vi "IVI_Oscilloscope.vi"() -> ()   [LabVIEW 2013]
doc: "This example shows how to use autosetup and acquire a waveform on a single channel for acquiring waveforms in a loop until stopped by user."
uses:
  IVI_chan.ctl
  Global.vi
panel:
  out "SQUID":string="24"
  in  "stop":bool
  in  "Tab Control":T1(tab)
  out "Saving":bool
  out "Waveform Data":waveform(dbl)[](graph)=[{"t0"=timestamp(1.3199999999947629e-08 s since 1904-01-01), "dt"=1e-06, "Y"=array[1000 elements]}, {"t0"=timestamp(1.3199999999947629e-08 s since 1904-01-01), "dt"=1e-06, "Y"=array[1000 elements]}]
  out "Points":i32=1000
  out "dt":dbl=1e-06 format="%#_2e"
  out "Repeat":u32=117
  out "Manufacturer":string="TEKTRONIX"
  out "Model":string="TDS 3054"
  out "Stats":T2(array[cluster])=[{"Min"=-2.081126189757815, "t (min)"=0.00037999999999999997, "Max"=3.0405276847871723, "t (max)"=0.0006399999999999999, "Range"=5.121653874544988, "Mean"=0.4992700288991155, "Std"=1.7686679103049028}, {"Min"=-1.0, "t (min)"=0.00030199999999999997, "Max"=1.0, "t (max)"=1.7e-05, "Range"=2.0, "Mean"=0.13208653234179343, "Std"=0.8981746888230542}] {"t (min)" format="%#_6p"; "t (max)" format="%#_6p"}
  in  "trigger level":dbl format="%#_13g"
  in  "trigger slope":i32(ring)=1 items=["Positive"=1, "Negative"=0]
  in  "trigger coupling":i32(ring)=1 items=["AC"=0, "DC"=1, "HF Reject"=3, "LF Reject"=4, "Noise Reject"=5]
  in  "trigger source":string(combo)="CHANNEL1"
  out "error out":errorcluster
  in  "Channels":T3[](array[typedef])=[{"channel name"="CHANNEL1", "probe attenuation"=1.0, "vertical offset"=0.0, "vertical range"=10.0, "vertical coupling"=1, "input impedance"=1000000.0}, {"channel name"="CHANNEL2", "probe attenuation"=1.0, "vertical offset"=0.0, "vertical range"=2.0, "vertical coupling"=1, "input impedance"=1000000.0}] {"input impedance" format="%#_13g"; "vertical coupling" items=["AC", "DC", "GND"]; "vertical range" format="%.3f"; "vertical offset" format="%.3f"; "probe attenuation" format="%.3f"}
  in  "logical name":refnum<k15>="Scope" caption="IVI Oscilloscope"
  in  "time per record":dbl=0.001 format="%^.2e"
  in  "acquisition start time":dbl format="%.3f"
  in  "min record length":i32=1000
  in  "wait (ms)":u32=500
  in  "Bin size":i16=1
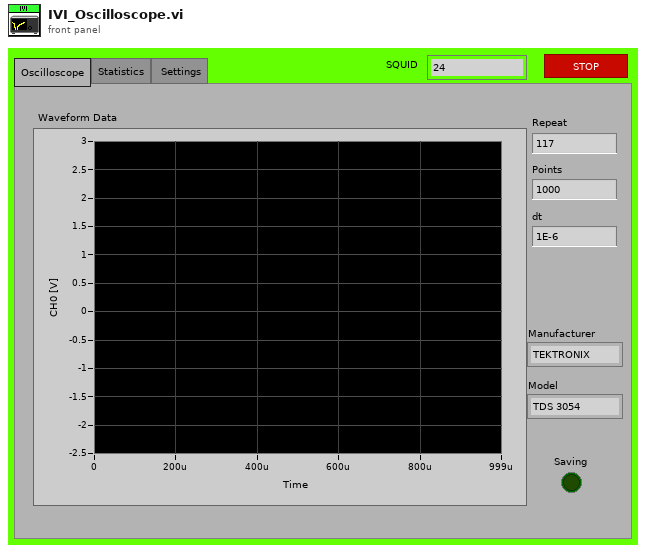
[diagram p1: front panel]
types:
  T1 = enum32{"Oscilloscope", "Statistics", " Settings"}
  T2 = cluster{"Min":dbl, "t (min)":dbl, "Max":dbl, "t (max)":dbl, "Range":dbl, "Mean":dbl, "Std":dbl}[]
  T3 = typedef "IVI_chan.ctl" = cluster{"channel name":string, "probe attenuation":dbl, "vertical offset":dbl, "vertical range":dbl, "vertical coupling":i32, "input impedance":dbl}
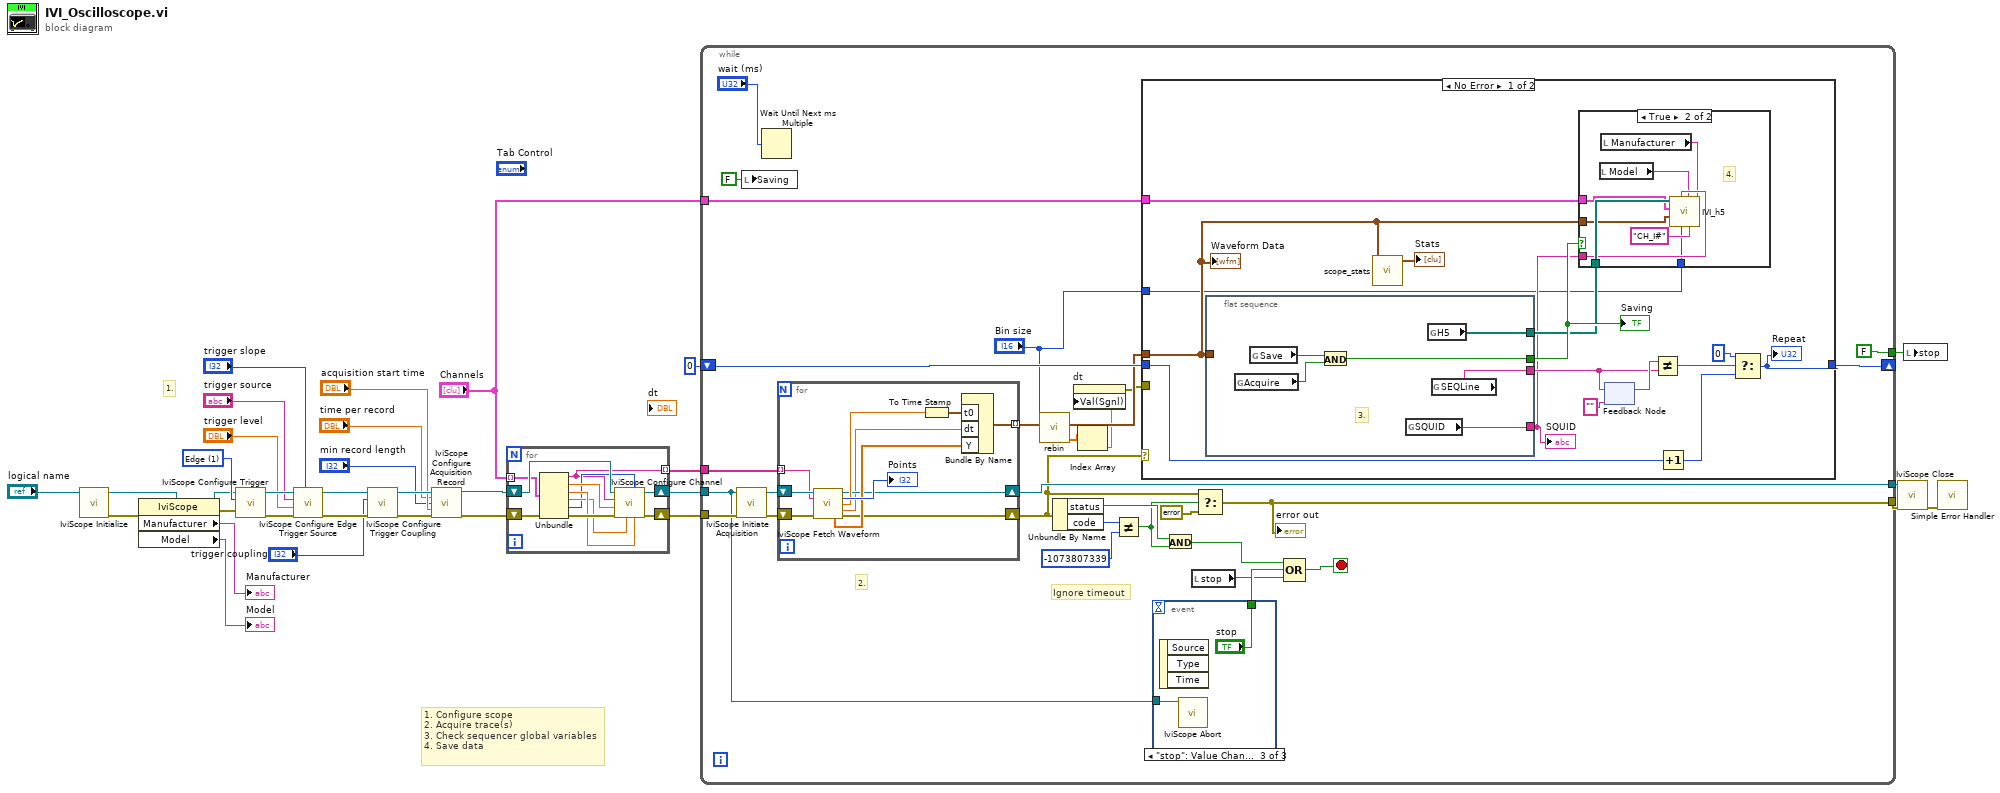
[diagram p0: block diagram]
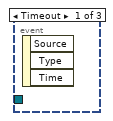
[diagram p2: hidden frame]
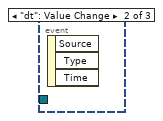
[diagram p3: hidden frame]
diagram:
  w29 = 1 items=["Edge"=1, "TV"=5, "Runt"=3, "Glitch"=4, "Width"=2, "AC Line"=7, "Immediate"=6] ("trigger type (Edge)")
  # "1."
  # "1. Configure scope\n2. Acquire trace(s)\n3. Check sequencer global variables\n4. Save data"
  n1 = call <vilib>:"IviScope Initialize.vi"("logical name (\"SampleScope\")"="logical name") -> ("error out"=w6:errorcluster, "instrument handle out"=w5:refnum<k15>)  [unwired: 9 in]
  n2 = property class="IviScope"(reference=w5, error in=w6) -> (reference out=w4:refnum<k15>, error out=w3:errorcluster, "Manufacturer"=→"Manufacturer":string, "Model"=→"Model":string)
  n3 = call <vilib>:"IviScope Configure Trigger.vi"("error in (no error)"=w3, "trigger type (Edge)"=w29, "instrument handle"=w4) -> ("error out"=w26:errorcluster, "instrument handle out"=w27:refnum<k15>)  [unwired: 7 in]
  n4 = call <vilib>:"IviScope Configure Edge Trigger Source.vi"("trigger slope (Positive)"="trigger slope", "error in (no error)"=w26, "trigger level  (0.0 V)"="trigger level", "trigger source (CHANNEL1)"="trigger source", "instrument handle"=w27) -> ("error out"=w25:errorcluster, "instrument handle out"=w28:refnum<k15>)  [unwired: 5 in]
  n5 = call <vilib>:"IviScope Configure Trigger Coupling.vi"("error in (no error)"=w25, "trigger coupling (DC)"="trigger coupling", "instrument handle"=w28) -> ("error out"=w24:errorcluster, "instrument handle out"=w23:refnum<k15>)  [unwired: 7 in]
  n6 = call <vilib>:"IviScope Configure Acquisition Record.vi"("instrument handle"=w23, "time per record (1.0E-3 s)"="time per record", "min record length (100 samples)"="min record length", "acquisition start time (0.0 s)"="acquisition start time", "error in (no error)"=w24) -> ("instrument handle out"=w20:refnum<k15>, "error out"=w21:errorcluster)  [unwired: 9 in]
  n7 = for {
    tunnel: "Channels" -> [w38] mode=indexing
    shift-right: [w42] -> w17
    shift-left: w20 -> [w39]
    shift-right: [w41] -> w16
    shift-left: w21 -> [w40]
    tunnel: [w33] -> w11 mode=indexing
    n8 = Unbundle(w38) -> ("channel name"=w33:string, "probe attenuation"=w37:dbl, "vertical offset"=w36:dbl, "vertical range"=w35:dbl, "vertical coupling"=w34:i32)  [unwired: 1 out]
    n9 = call <vilib>:"IviScope Configure Channel.vi"("vertical offset (0.0 V)"=w36, "vertical coupling (DC)"=w34, "vertical range (10.0 V)"=w35, "error in (no error)"=w40, "probe attenuation (1:1.0)"=w37, "channel name (\"CHANNEL1\")"=w33, "instrument handle"=w39) -> ("error out"=w41:errorcluster, "instrument handle out"=w42:refnum<k15>)  [unwired: 3 in]
  }
  n10 = while {
    tunnel: [w56] -> w10
    tunnel: [w63] -> w8
    shift-right: [w65] -> _
    shift-left: u32 0 ("millisecond multiple") -> [w66]
    tunnel: [FALSE ("stop")] -> w31
    tunnel: w17 -> [w52]
    tunnel: w16 -> [w60]
    tunnel: w11 -> [w57]
    tunnel: "Channels" -> [w54]
    stop <- w70 stop-if-true
    # "Ignore timeout"
    # "2."
    n11 = call <vilib>:"IviScope Initiate Acquisition.vi"("error in (no error)"=w60, "instrument handle"=w52) -> ("error out"=w58:errorcluster, "instrument handle out"=w59:refnum<k15>)  [unwired: 8 in]
    n12 = local write "Saving"(FALSE ("Saving")) -> ()
    n13 = Wait Until Next ms Multiple(millisecond multiple="wait (ms)") -> ()  [unwired: 1 out]
    n14 = for {
      tunnel: w57 -> [w81] mode=indexing
      tunnel: [w77] -> w47 mode=indexing
      shift-right: [w76] -> w56
      shift-left: w59 -> [w83]
      shift-right: [w74] -> w55
      shift-left: w58 -> [w84]
      n15 = call <vilib>:"IviScope Fetch Waveform.vi"("instrument handle"=w83, "channel name (\"CHANNEL1\")"=w81, "error in (no error)"=w84) -> ("instrument handle out"=w76:refnum<k15>, "actual points"=→"Points":i32, "initial x"=w78:dbl, "x increment"=w75:dbl, "waveform array"=w80:dbl[], "error out"=w74:errorcluster)  [unwired: 7 in]
      n16 = To Time Stamp(1:w78) -> (0:w79:timestamp)
      n17 = Bundle By Name("t0"=w79, "dt"=w75, "Y"=w80) -> (w77:waveform(dbl))  [unwired: 1 in]
    }
    n18 = call "rebin.vi"("Bin size"="Bin size", "Waveform Data IN"=w47) -> ("dt"=w45:dbl[], "Waveform Data OUT"=w48:waveform(dbl)[])  [unwired: 6 in, 1 out]
    n19 = Unbundle By Name(w55) -> ("status"=w67:bool, "code"=w69:i32)
    n20 = Index Array(array=w45) -> (element=w46:dbl)  [unwired: 1 in]
    n21 = property on="dt" class="DigNum (strict)"("Val(Sgnl)"=w46) -> (error out=w44:errorcluster)  [unwired: 2 in, 1 out]
    n22 = Not Equal?(x=w69, y=-1073807339) -> (x != y?=w64:bool)
    n23 = case shown="No Error" w55 {
      tunnel: w48 -> [w92 _]
      tunnel: w66 -> [w95 w114]
      tunnel: [w89 w114] -> w65
      tunnel: w54 -> [w91 _]
      tunnel: w44 -> [_ _]
      tunnel: "Bin size" -> [w85 _]
      frame No Error {
        n24 = flat-sequence {
          tunnel: w92 -> [_]
          tunnel: [w103] -> w90
          tunnel: [w102] -> w88
          tunnel: [w101] -> w87
          tunnel: [w100] -> w86
          frame #0 {
            # "3."
            n25 = global read "Global.vi" "Acquire"() -> (w105:bool)
            n26 = global read "Global.vi" "Save"() -> (w104:bool)
            n27 = And(x=w104, y=w105) -> (x .and. y?=w103:bool)
            n28 = global read "Global.vi" "SQUID"() -> (w100:string)
            n29 = global read "Global.vi" "H5"() -> (w101:path[])
            n30 = global read "Global.vi" "SEQLine"() -> (w102:string)
          }
        }
        n31 = call "scope_stats.vi"("Waveform Data"=w92) -> ("Stats"=→"Stats":T2)  [unwired: 7 in]
        n32 = case shown="True" w90 {
          tunnel: w92 -> [_ w112]
          tunnel: w91 -> [_ w109]
          tunnel: w87 -> [_ w113]
          tunnel: w86 -> [_ w111]
          tunnel: w85 -> [_ w106]
          frame False {
          }
          frame True {
            # "4."
            n33 = local read "Model"() -> (w107:string)
            n34 = local read "Manufacturer"() -> (w108:string)
            n35 = call "IVI_h5.vi"("Model"=w107, "TYPE"="CH_I#", "Manufacturer"=w108, "Bin size"=w106, "SQUID"=w111, "Waveform Data"=w112, "Channels"=w109, "H5"=w113) -> ()  [unwired: 3 in, 1 out]
          }
        }
        n36 = feedback #1("" ("Seq")) -> (w98:string)
        n37 = feedback-in #1(w88) -> ()
        n38 = Not Equal?(x=w98, y=w88) -> (x != y?=w94:bool)
        n39 = Increment(x=w95) -> (x+1=w96:u32)
        n40 = Select(t=u32 0, s=w94, f=w96) -> (s? t:f=w89:u32)
        "Repeat" <- w89
        "Waveform Data" <- w92
        "Saving" <- w90
        "SQUID" <- w86
      }
      frame Error {
      }
    }
    n41 = event shown="[2] \"stop\": Value Change" {
      selector: _ -> [_ _ _]
      dyn-events: _ -> [_ _ _]
      timeout: _ -> [_ _ _]
      tunnel: [_ _ "stop"] -> w53
      tunnel: w52 -> [_ _ w72]
      event Timeout {
        n42 = event-data() -> ()  [unwired: 1 in, 3 out]
      }
      event "dt": Value Change {
        n43 = event-data() -> ()  [unwired: 1 in, 3 out]
      }
      event "stop": Value Change {
        n44 = event-data() -> ()  [unwired: 1 in, 3 out]
        n45 = call <vilib>:"IviScope Abort.vi"("instrument handle"=w72) -> ()  [unwired: 9 in, 2 out]
      }
    }
    n46 = And(x=w67, y=w64) -> (x .and. y?=w51:bool)
    n47 = local read "stop"() -> (w50:bool)
    n48 = Select(t=w55, s=w64, f=errorcluster {"status"=FALSE, "code"=0, "source"=""} ("error out")) -> (s? t:f=w63:errorcluster)
    "error out" <- w63
    n49 = Compound Arithmetic op=OR(w51, w53, w50) -> (w70:bool)
  }
  n50 = call <vilib>:"IviScope Close.vi"("error in (no error)"=w8, "instrument handle"=w10) -> ("error out"=w9:errorcluster)  [unwired: 9 in]
  n51 = local write "stop"(w31) -> ()
  n52 = call <vilib>:"Simple Error Handler.vi"("error in (no error)"=w9) -> ()  [unwired: 4 in, 5 out]
